vi "CustomErrorFG.vi"(9 "Custom description in":string caption="Custom description in (\"\")", 10 "Custom code":i32, 11 "Function":T1) -> (1 "Custom descriptions out":string[](array[string]), 2 "Custom code found?":bool)   [LabVIEW 2017, in "GPError.lvlib"]
doc: "FG containing the custom error/warning code definitions for this LabVIEW instance.\n\n<B>Custom description in</B> is only used when <B>Function</B> is 'Set custom code'. If the custom code has already been set, the existing description will only be overwritten if <B>Custom description in</B> is not an empty string.\n\nSteen Schmidt\nGPower\n25/12 2011"
uses:
  GPError.lvlib
  CustomDescriptions.ctl
  CustomErrorFGFunction.ctl
panel:
  # "Copyright © 2013\nSteen Schmidt, GPower\nSee enclosed license file for terms and conditions"
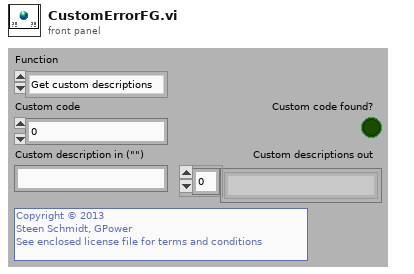
[diagram p1: front panel]
types:
  T1 = typedef "GPError.lvlib/CustomErrorFGFunction.ctl" = enum16{"Get custom descriptions", "Set custom code", "Unset custom code"}
  T2 = typedef "GPError.lvlib/CustomDescriptions.ctl" = cluster{"Descriptions":string[]}
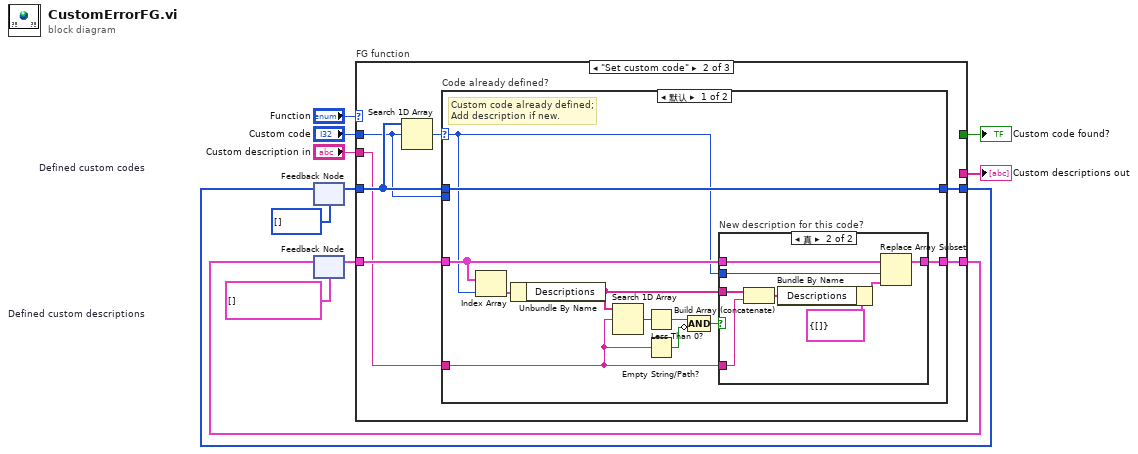
[diagram p0: block diagram]
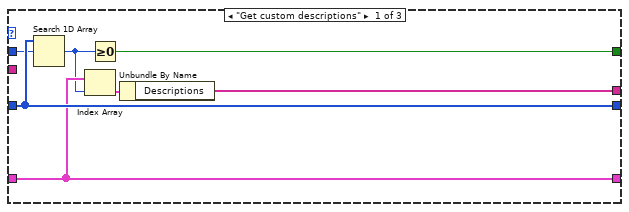
[diagram p2: hidden frame]
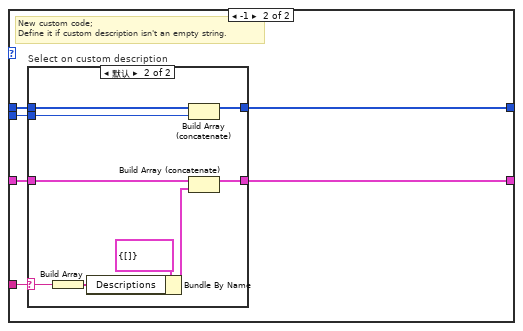
[diagram p4: hidden frame]
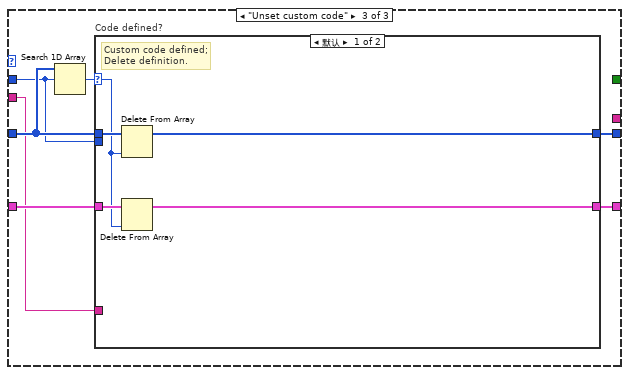
[diagram p6: hidden frame]
diagram:
  n1 = feedback #1 "Defined custom codes"(i32[] [] ("Defined custom error codes")) -> (w9:i32[])
  n2 = feedback #2 "Defined custom descriptions"(T2[] []) -> (w8:T2[])
  n3 = case "FG function" shown="\"Set custom code\"" "Function" {
    tunnel: "Custom description in" -> [_ w20 w64]
    tunnel: "Custom code" -> [w17 w19 w63]
    tunnel: w9 -> [w18 w25 w69]
    tunnel: w8 -> [w15 w24 w68]
    tunnel: [w18 w23 w67] -> w5
    tunnel: [w15 w22 w66] -> w6
    tunnel: [w16 _ _] -> w7
    tunnel: [w12 _ _] -> w1
    frame "Get custom descriptions" {
      n4 = Search 1D Array(1D array=w18, element=w17) -> (index of element=w14:i32)  [unwired: 1 in]
      n5 = Index Array(array=w15, index=w14) -> (element=w13:T2)
      n6 = Greater Or Equal To 0?(x=w14) -> (x >= 0?=w16:bool)
      n7 = Unbundle By Name(w13) -> ("Descriptions"=w12:string[])
    }
    frame "Set custom code" {
      n8 = Search 1D Array(1D array=w25, element=w19) -> (index of element=w21:i32)  [unwired: 1 in]
      n9 = case "Code already defined?" shown="默认" w21 {
        selector: w21 -> [w33 _]
        tunnel: w25 -> [w36 w51]
        tunnel: w24 -> [w34 w48]
        tunnel: [w36 w49] -> w23
        tunnel: [w35 w47] -> w22
        tunnel: w19 -> [_ w50]
        tunnel: w20 -> [w26 w46]
        frame Default {
          # "Custom code already defined;\nAdd description if new."
          n10 = Index Array(array=w34, index=w33) -> (element=w32:T2)
          n11 = Unbundle By Name(w32) -> ("Descriptions"=w27:string[])
          n12 = Search 1D Array(1D array=w27, element=w26) -> (index of element=w31:i32)  [unwired: 1 in]
          n13 = Less Than 0?(x=w31) -> (x < 0?=w30:bool)
          n14 = Empty String/Path?(string/path=w26) -> (empty?=w29:bool)
          n15 = Compound Arithmetic op=AND(w30, invert w29) -> (w28:bool)
          n16 = case "New description for this code?" shown="真" w28 {
            tunnel: w34 -> [w37 w45]
            tunnel: [w37 w44] -> w35
            tunnel: w33 -> [_ w43]
            tunnel: w27 -> [_ w42]
            tunnel: w26 -> [_ w41]
            frame False {
            }
            frame True {
              n17 = Build Array (concatenate)(w42, w41) -> (w39:string[])
              n18 = Bundle By Name(cluster=T2 {"Descriptions"=[]} ("Descriptions"), "Descriptions"=w39) -> (w38:T2)
              n19 = Replace Array Subset(array=w45, new element=w38, index=w43) -> (w44:T2[])
            }
          }
        }
        frame -1 {
          # "New custom code;\nDefine it if custom description isn't an empty string."
          n20 = case "Select on custom description" shown="默认" w46 {
            selector: w46 -> [_ w56]
            tunnel: w51 -> [w53 w62]
            tunnel: w50 -> [_ w61]
            tunnel: [w53 w60] -> w49
            tunnel: w48 -> [w52 w59]
            tunnel: [w52 w58] -> w47
            frame "" {
              # "Empty string;\nDon't set custom description."
            }
            frame Default {
              n21 = Build Array(w56) -> (w55:string[])
              n22 = Bundle By Name(cluster=T2 {"Descriptions"=[]} ("Descriptions"), "Descriptions"=w55) -> (w54:T2)
              n23 = Build Array (concatenate)(w62, w61) -> (w60:i32[])
              n24 = Build Array (concatenate)(w59, w54) -> (w58:T2[])
            }
          }
        }
      }
    }
    frame "Unset custom code" {
      n25 = Search 1D Array(1D array=w69, element=w63) -> (index of element=w65:i32)  [unwired: 1 in]
      n26 = case "Code defined?" shown="默认" w65 {
        selector: w65 -> [w72 _]
        tunnel: w69 -> [w74 w76]
        tunnel: w68 -> [w73 w75]
        tunnel: [w71 w76] -> w67
        tunnel: [w70 w75] -> w66
        tunnel: w63 -> [_ _]
        tunnel: w64 -> [_ _]
        frame Default {
          # "Custom code defined;\nDelete definition."
          n27 = Delete From Array(array=w74, index=w72) -> (array with subset deleted=w71:i32[])  [unwired: 1 in, 1 out]
          n28 = Delete From Array(array=w73, index=w72) -> (array with subset deleted=w70:T2[])  [unwired: 1 in, 1 out]
        }
        frame -1 {
          # "Custom code not defined;\nDone."
        }
      }
    }
  }
  "Custom code found?" <- w7
  "Custom descriptions out" <- w1
  n29 = feedback-in #1(w5) -> ()
  n30 = feedback-in #2(w6) -> ()
